vi "script vstand model UI.vi"() -> ()   [LabVIEW 2014, in "CD model script.lvlib"]
uses:
  CD model script.lvlib
panel:
  in  "release/debug?":bool
  in  "build?":bool
  in  "run":bool
  in  "Model VI path":path
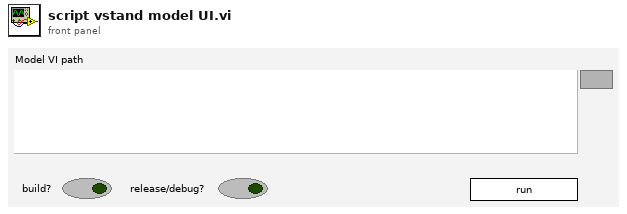
[diagram p1: front panel]
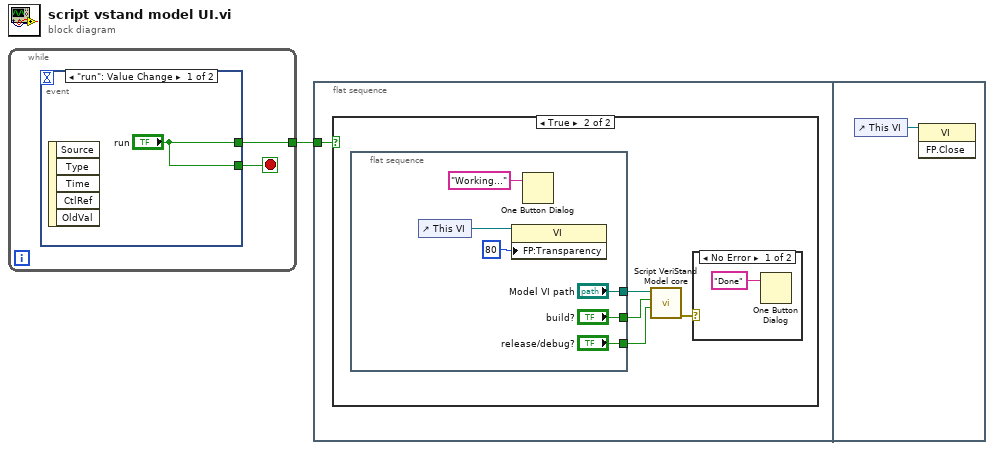
[diagram p0: block diagram]
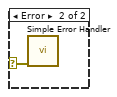
[diagram p3: hidden frame]
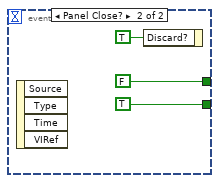
[diagram p4: hidden frame]
diagram:
  n1 = while {
    tunnel: [w2] -> w1
    stop <- w3 stop-if-true
    n2 = event shown="[0] \"run\": Value Change" {
      selector: _ -> [_ _]
      dyn-events: _ -> [_ _]
      timeout: _ -> [_ _]
      tunnel: ["run" TRUE ("Discard?")] -> w3
      tunnel: ["run" FALSE ("run")] -> w2
      event "run": Value Change {
        n3 = event-data() -> ()  [unwired: 1 in, 5 out]
      }
      event Panel Close? {
        n4 = event-data() -> ()  [unwired: 1 in, 4 out]
        n5 = event-data("Discard?"=TRUE) -> ()  [unwired: 1 in, 1 out]
      }
    }
  }
  n6 = flat-sequence {
    tunnel: w1 -> [w8]
    frame #0 {
      n7 = case shown="True" w8 {
        frame False {
        }
        frame True {
          n8 = flat-sequence {
            tunnel: ["build?"] -> w11
            tunnel: ["release/debug?"] -> w10
            tunnel: ["Model VI path"] -> w9
            frame #0 {
              n9 = control-ref of="This VI"() -> (w14:refnum<vi>)
              n10 = property class="VI"(reference=w14, "FP:Transparency"=u8 80 ("Front Panel Window:Transparency")) -> ()  [unwired: 1 in, 2 out]
              n11 = One Button Dialog(message="Working...") -> ()  [unwired: 1 in, 1 out]
            }
          }
          n12 = call "Script VeriStand Model core.vi"("release/debug?"=w10, "build?"=w11, "VI path"=w9) -> ("error out"=w12:errorcluster)  [unwired: 8 in]
          n13 = case shown="No Error" w12 {
            selector: w12 -> [_ w20]
            frame No Error {
              n14 = One Button Dialog(message="Done") -> ()  [unwired: 1 in, 1 out]
            }
            frame Error {
              n15 = call <vilib>:"Simple Error Handler.vi"("error in (no error)"=w20) -> ()  [unwired: 4 in, 5 out]
            }
          }
        }
      }
    }
    frame #1 {
      n16 = control-ref of="This VI"() -> (w21:refnum<vi>)
      n17 = invoke class="VI" method="FP.Close"(reference=w21) -> ()  [unwired: 2 in, 3 out]
    }
  }
